vi "SVF System Simplified.vi"() -> ()   [LabVIEW 2012]
uses:
  <vilib>/addons/Control Design/_Model Construction/Data Typedefs.llb/CD Model Type.ctl
  <vilib>/addons/Control Design/_Model Construction/Model Typedefs.llb/CD Zero-Pole-Gain Model (MIMO).ctl
  <vilib>/addons/Control Design/_Model Construction/Model Typedefs.llb/CD General Elements.ctl
  <vilib>/addons/Control Design/_Model Construction/Model Typedefs.llb/CD Zero-Pole-Gain Model (SISO).ctl
  <vilib>/Simulation/Scripting/Companion Diagram/SimConfigNode/SimParams.ctl
  <vilib>/Simulation/Scripting/Companion Diagram/SimConfigNode/_simSolvers.ctl
  <vilib>/Simulation/Implementation/Shared/SIMSCR Execution Mode.ctl
  <vilib>/Platform/TimedLoop/XDataNode/timing_clust.ctl
  <vilib>/Platform/TimedLoop/XDataNode/nitl_modes.ctl
  <vilib>/Platform/TimedLoop/XDataNode/wakeup.ctl
  <vilib>/Simulation/Param Hierarchy/Typedefs/SIMPH Param Control Actions.ctl
  <vilib>/Simulation/Scripting/Editor Utilities/SIM subVI tag data.ctl
  <vilib>/Simulation/Scripting/Editor Utilities/SIM subVI execution type.ctl
  <vilib>/Simulation/Implementation/Shared/NILVSim_ParamChanged.vi
  <vilib>/Simulation/Implementation/Shared/NILVSim_FinishedLate.vi
  <vilib>/Simulation/ContinuousLinear/Implementation/NILVSim State Space.llb/SIM State Space Distributor (CD).vi
  <vilib>/Simulation/ContinuousLinear/Implementation/NILVSim Derivative.llb/SIM derivative (scalar).vi
  <vilib>/Simulation/ContinuousLinear/Implementation/NILVSim Transfer Function.llb/SIM Transfer Function Distributor (SISO).vi
  <vilib>/Simulation/ContinuousLinear/Implementation/NILVSim Transfer Function.llb/SIM Transfer Function Collector (SISO).vi
  <vilib>/Simulation/SignalDisplay/Implementation/NILVSim Time Waveform.llb/SIM Time Waveform (vector).vi
  <vilib>/Simulation/ContinuousLinear/Implementation/NILVSim State Space.llb/SIM State Space Collector (CD).vi
  <vilib>/Simulation/Implementation/Shared/SIM Fire Discrete SubVI.vi
  <vilib>/Simulation/Utility/Implementation/SIM Halt.vi
  <vilib>/Simulation/Implementation/Shared/NILVSim_Manager.vi
  <vilib>/Simulation/Implementation/Shared/NILVSim_FinalizeModel.vi
  <vilib>/Simulation/SignalArithmetic/Implementation/NILVSim Gain.llb/SIM Gain (scalar).vi
  <vilib>/Simulation/DiscreteLinear/Implementation/NILVSim Discrete State Space Buffered.llb/SIM Discrete State Space Distributor (CD).vi
  <vilib>/Simulation/SignalArithmetic/Implementation/NILVSim Gain.llb/SIM Gain (vector).vi
  <vilib>/Simulation/DiscreteLinear/Implementation/NILVSim Discrete State Space Buffered.llb/SIM Discrete State Space Collector (CD).vi
  <vilib>/Simulation/Implementation/Shared/SIM Fire Discrete SubVI (Core).vi
  <vilib>/addons/Control Design/_Dynamic Analysis/Dynamic Analysis.llb/Dynamic Analysis subVI/cd_Pole-Zero Map (State-Space).vi
  <vilib>/addons/Control Design/_Model Conversions/Model Type.llb/Model Conversion SubVI/cd_Convert State-Space to Zero-Pole-Gain Model.vi
  <vilib>/addons/Control Design/_Model Construction/Model Information.llb/Model Information SubVIs/cd_Verify If Discrete (State-Space).vi
  <vilib>/addons/Control Design/_Model Construction/Model Information.llb/Model Information SubVIs/cd_Check State Space Model.vi
  <vilib>/addons/Control Design/_Model Construction/Model Information.llb/Model Information SubVIs/cd_Verify Model Type (SS).vi
  <vilib>/addons/Control Design/_Dynamic Analysis/Dynamic Analysis.llb/Dynamic Analysis subVI/cd_Poles (State-Space).vi
  <vilib>/addons/Control Design/_Model Construction/Model Creation.llb/Model Creation SubVI/cd_Create State Space Model.vi
  <vilib>/addons/Control Design/_Model Conversions/Continuous and Discrete.llb/Continuous and Discrete SubVI/cd_Convert Continuous to Discrete (SS).vi
  <vilib>/Simulation/Implementation/Shared/SIM Unbundle Sim Info.vi
  <vilib>/Utility/error.llb/Clear Errors.vi
  <vilib>/Simulation/Implementation/Shared/NILVSim_GetModelError.vi
  <vilib>/Simulation/Implementation/Shared/SIM Bundle Sim Info.vi
  <vilib>/Simulation/Implementation/Shared/SIMSH Read Queue.vi
  <vilib>/Simulation/Implementation/Shared/NILVSim_Initialize.vi
  <vilib>/addons/Control Design/_Implementation/CD State Feedback Controller.vi
  <vilib>/addons/Control Design/_Implementation/CD State Feedback Controller (Single Output).vi
  <vilib>/Simulation/Utility/Implementation/NILVSim Get Time and IsAcceptedStep.vi
  Program Files/National Instruments/LabVIEW 2012/examples/Control and Simulation/Case Studies/Mechatronics/Inverted Pendulum/subVIs/Draw Linear Inverted Pendulum_sim.vi
  <vilib>/Simulation/Scripting/Companion Diagram/SimConfigNode/SimDog.xnode
  <vilib>/Platform/TimedLoop/XDataNode/XDataNode.xnode
  <vilib>/Simulation/Implementation/XNodeFramework/SimXNode/SimX.xnode
  <vilib>/addons/Control Design/_Implementation/NI_CD_Implementation.lvlib
  <vilib>/Simulation/ContinuousLinear/Implementation/NILVSim Transfer Function.llb/SIM Transfer Function (SISO).vi
  <vilib>/addons/Control Design/_Model Construction/NI_LinSys_Model Typedefs.lvlib
  <vilib>/addons/Control Design/_Model Construction/Model Typedefs.llb/CD State Space Model (MIMO).ctl
  <vilib>/Simulation/ContinuousLinear/Implementation/NILVSim State Space.llb/SIM State Space (CD).vi
  <vilib>/addons/Control Design/_State Feedback Control/NI_CD_State Feedback Control.lvlib
  <vilib>/addons/Control Design/_Model Construction/NI_LinSys_Model Creation.lvlib
  <vilib>/addons/Control Design/_Dynamic Analysis/NI_CD_Dynamic Analysis.lvlib
  <vilib>/addons/Control Design/_Model Conversions/NI_CD_Continuous and Discrete.lvlib
  <vilib>/addons/Control Design/_State-Space Analysis/NI_CD_State-Space Analysis.lvlib
  <vilib>/addons/Control Design/_Model Construction/NI_LinSys_Model Information.lvlib
  <vilib>/addons/Control Design/_Model Conversions/NI_CD_Model Type.lvlib
  <vilib>/Platform/TimedLoop/XDataNode/XDNodeRunTimeDep.lvlib
  <vilib>/Simulation/Implementation/Shared/NI_SIM_Implementation.lvlib
  <vilib>/Simulation/DiscreteLinear/Implementation/NILVSim Discrete State Space Buffered.llb/SIM Discrete State Space Buffered (CD).vi
  <vilib>/addons/Control Design/_Model Construction/NI_LinSys_Data Typedefs.lvlib
panel:
  in  "Input Signal (IMU)":dbl(slide) scale=0.0..10.0
  out "Controller Gain":dbl[](array[numeric])
  out "Waveform Plot":waveform(dbl)[](graph)
  in  "Inertia of pendulum (I)":dbl
  in  "Length to center of mass (l)":dbl
  in  "Kinetic friction of robot (b)":dbl
  in  "Mass of Rest (m)":dbl
  in  "Mass of Bottom Wheel (M)":dbl
  out "Pole-Zero Map":cluster{dbl[], dbl[]}[](graph)
  out "Zero-Pole-Gain Model":T1 {"zero-pole-gain(s)"."delay" format="%.4f"; "zero-pole-gain(s)"."Poles" format="%#.8g"; "zero-pole-gain(s)"."Zeros" format="%#.8g"; "zero-pole-gain(s)"."Gain" format="%#.8g"; "properties"."Sampling Time" format="%#.6p"; "properties"."Output Delays" format="%.4f"; "properties"."Input Delays" format="%.4f"}
  out "Static Gain Case?":bool
  out "Type of Model":T4 items=["Empty", "SISO", "SIMO", "MISO", "MIMO", "Undetermined"]
  out "Number of Outputs":i32
  out "Number of Inputs":i32
  out "Number of States":i32
  out "Sampling Time Required":dbl format="%.2f"
  out "Discrete?":bool
  out "Controllability Matrix":dbl[][](array[numeric])=[[1.0, 0.0, 6.0], [0.0, 1.0, -1.0], [0.0, 0.0, 0.0]] format="%.2f"
  out "Outputs":dbl[](array[numeric])
  out "Plot X and Theta":waveform(dbl)[](graph)=[{"t0"=timestamp(4.71 s since 1904-01-01), "dt"=1.0, "Y"=[-0.13996665083491025]}, {"t0"=timestamp(4.71 s since 1904-01-01), "dt"=1.0, "Y"=[-1.62298383744272e-05]}]
  in  "stop":bool
  in  "Tab Control":T5(tab)=enum."Controller"
  out "System Poles":cdb[](array[numeric])=[5.56510798020132+0.0i, -5.60409024766489+0.0i, -0.1428177325364319+0.0i, 0.0+0.0i] format="%#.2g"
  in  "Desired Poles":cdb[](array[numeric])=[-5.0+0.0i, -5.0+0.0i, -20.0+0.0i, -15.0+0.0i] format="%#.2g"
  out "Calculated Poles":cdb[](array[numeric])=[-19.999999999997662+0.0i, -15.000000000017264+0.0i, -4.999999999995586+4.2610378298679e-06i, -4.999999999995586-4.2610378298679e-06i] format="%#.2g"
  in  "Initial Conditions":T6
  in  "Set Point (m)":dbl(slide)=-0.14 scale=-0.2..0.2
  out "Feedback Gain (K)":dbl[](array[numeric])=[-168.36531967948676, -87.08873750117637, 222.70457028739702, 44.69540040141787]
  out "Boundary Reached":bool
  in  "Discrete Mode":bool=TRUE
  in  "A":dbl[][](array[numeric])=[[0.0, 1.0, 0.0, 0.0], [0.0, -0.1818, 2.6727, 0.0], [0.0, 0.0, 0.0, 1.0], [0.0, -0.4545, 31.1818, 0.0]] format="%#.2g"
  in  "B":dbl[][](array[numeric])=[[0.0], [1.8182], [0.0], [4.5455]] format="%#.2g"
  in  "C":dbl[][](array[numeric])=[[1.0, 0.0, 0.0, 0.0], [0.0, 0.0, 1.0, 0.0]] format="%#.2g"
  in  "D":dbl[][](array[numeric])=[[0.0], [0.0]] format="%#.2g"
  in  "Sampling Time (s)":dbl=0.1
  out "3D Picture Control":refnum<vi>(3d-picture)
  # "MODEL INFO"
  # "DISCRETE INFO"
  # "If you installed the LabVIEW Control Design Toolkit, you can design a controller by specifying the locations of the Desired Poles.\n\nOtherwise, click the Controller tab to specify the controller Feedback Gain."
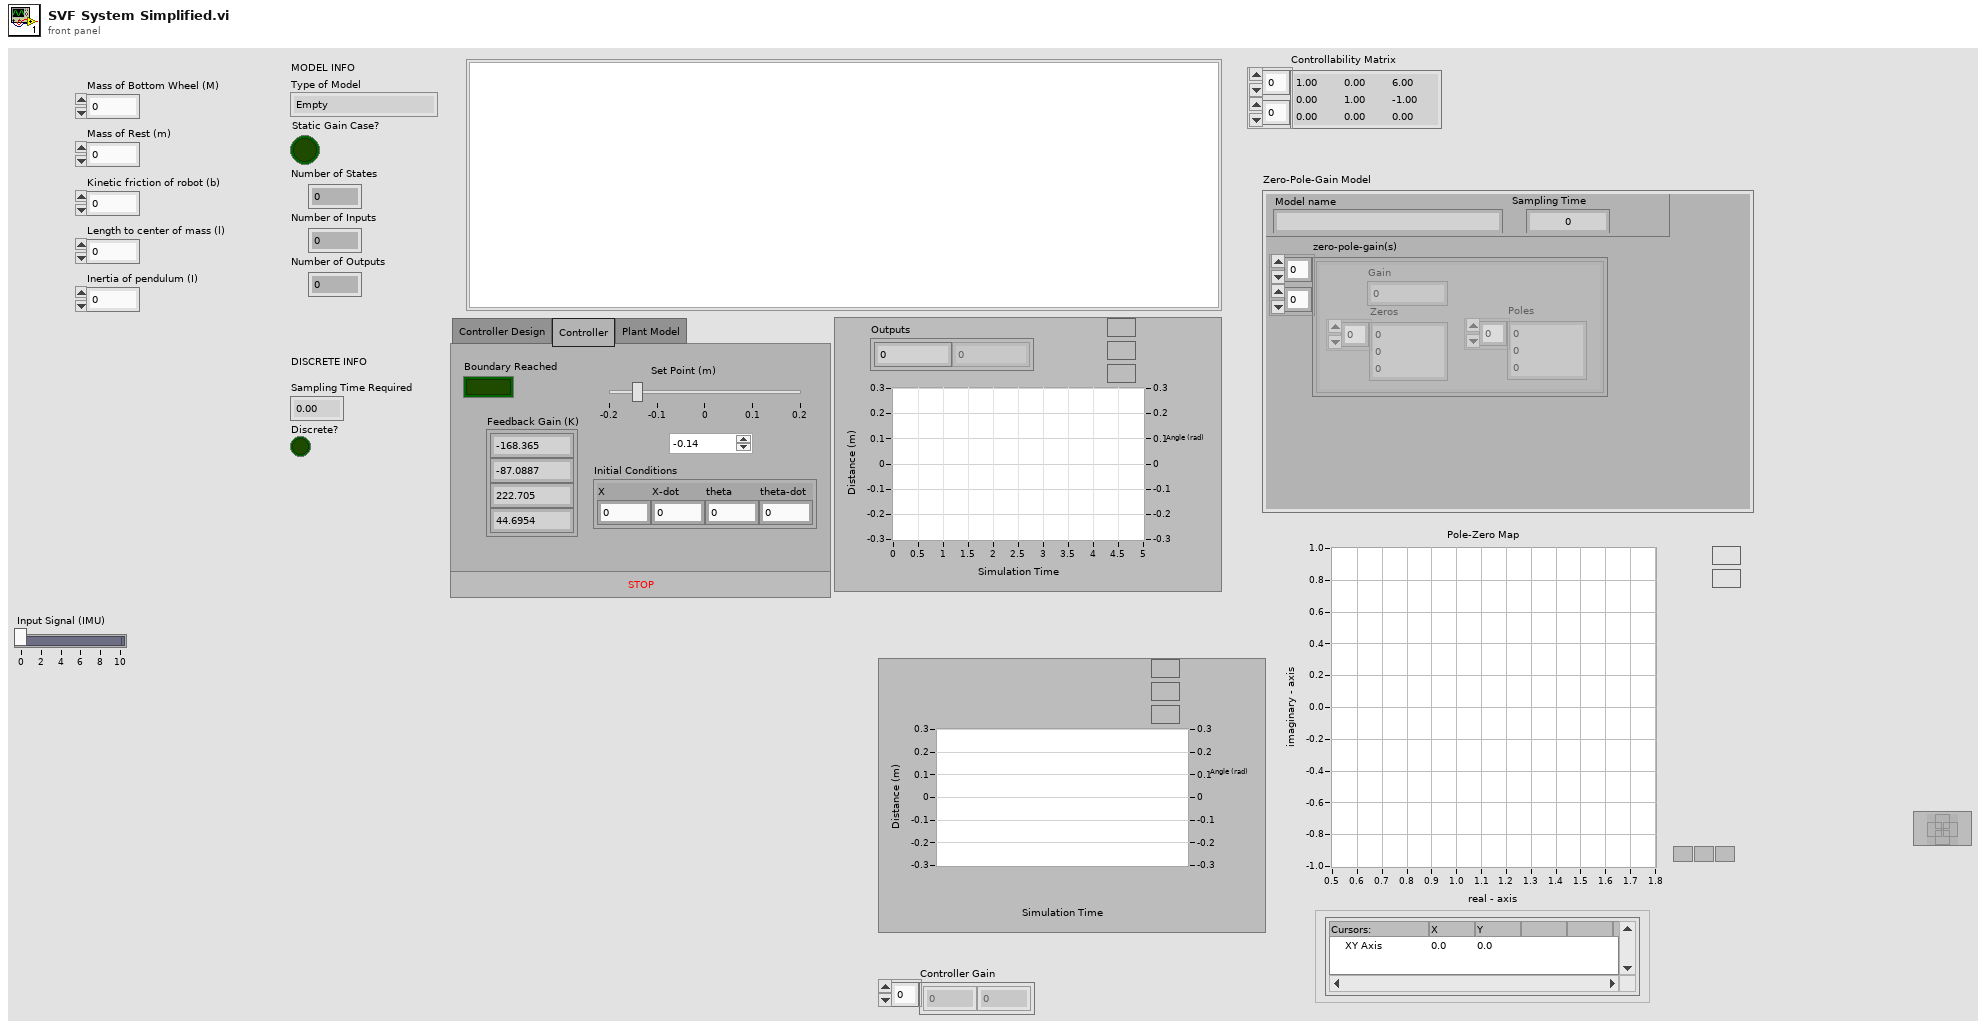
[diagram p1: front panel]
types:
  T1 = typedef "NI_LinSys_Model Typedefs.lvlib/CD Zero-Pole-Gain Model (MIMO).ctl" = cluster{"properties":T2, "zero-pole-gain(s)":T3[][]}
  T2 = typedef "NI_LinSys_Model Typedefs.lvlib/CD General Elements.ctl" = cluster{"Model name":string, "Input names":string[], "Output names":string[], "Input Delays":dbl[], "Output Delays":dbl[], "Sampling Time":dbl, "Notes":string}
  T3 = typedef "NI_LinSys_Model Typedefs.lvlib/CD Zero-Pole-Gain Model (SISO).ctl" = cluster{"Gain":dbl, "Zeros":cdb[], "Poles":cdb[], "delay":dbl}
  T4 = typedef "NI_LinSys_Data Typedefs.lvlib/CD Model Type.ctl" = u16
  T5 = enum32{"Controller Design", "Controller", "Plant Model"}
  T6 = cluster{"X":dbl, "X-dot":dbl, "theta":dbl, "theta-dot":dbl}
  T7 = typedef "NI_LinSys_Model Typedefs.lvlib/CD State Space Model (MIMO).ctl" = cluster{"properties":T2, "A":dbl[][], "B":dbl[][], "C":dbl[][], "D":dbl[][], "StateNames":string[], "Transport Delay":dbl[][]}
  T8 = typedef "SIMSCR Execution Mode.ctl" = enum16{"Simulate to Completion", "Single Time-Step Simulation (Fixed Step Only)"}
  T9 = typedef "XDNodeRunTimeDep.lvlib/timing_clust.ctl" = cluster{"Expected End [f-1]":u64, "Actual End [f-1]":u64, "Finished Late? [f-1]":bool, "Expected End [i-1]":u64, "Actual End [i-1]":u64, "Finished Late? [i-1]":bool, "Expected Start [i]":u64, "Actual Start [i]":u64, "Expected Start [f]":u64, "Actual Start [f]":u64, "Source Name":string, "Structure Name":string, "Period":i64, "Deadline":i64, "Offset":i64, "Start":i64, "Priority":i32, "Timeout":i32, "Mode":T10, "Wakeup Reason":T11, "Error":errorcluster, "Source Type":string, "Secondary Source Type":string, "Global End Time":u64, "Global Start Time":u64, "Frame Duration":u64, "Iteration Duration":u64, "Assigned CPU":i32, "I/O Scan Engine Mode":u32}
  T10 = typedef "XDNodeRunTimeDep.lvlib/nitl_modes.ctl" = enum32{"No Change", "Process missed periods, maintain original phase", "Discard missed periods, maintain original phase", "Process missed periods, ignore original phase", "Discard missed periods, ignore original phase"}
  T11 = typedef "XDNodeRunTimeDep.lvlib/wakeup.ctl" = enum32{"Normal", "Aborted", "Asynchronous wakeup", "Timing source error", "Timed loop error", "Timeout"}
  T12 = typedef "SIMPH Param Control Actions.ctl" = enum16{"get params", "set params"}
  T13 = typedef "SIM subVI tag data.ctl" = cluster{"period":dbl, "skew":dbl, "Simulation execution type":T14}
  T14 = typedef "SIM subVI execution type.ctl" = enum16{"Function call", "Discrete", "Continuous", "Initialization only", "Final step only"}
  T15 = typedef "SimParams.ctl" = cluster{"Initial Time (s)":dbl, "Final Time (s)":dbl, "Step Size (s)":dbl, "ODE Solver":T16, "Minimum Step Size (s)":dbl, "Maximum Step Size (s)":dbl, "Relative Tolerance":dbl, "Absolute Tolerance":dbl, "Software Timing":bool, "Initial Step Size (s)":dbl, "Automatic Fixed Step Size?":bool, "Automatic Discrete Step Size?":bool, "Discrete Step Size (s)":dbl, "Calculate using Time Step":bool, "Solver Wired?":bool, "Prev.Frm.Expected End":u64, "Prev.Frm.Actual End":u64, "Prev.Frm.Finished Late?":bool, "Prev.Iter.Expected End":u64, "Prev.Iter.Actual End":u64, "Prev.Iter.Finished Late?":bool, "Expected Iteration Start":u64, "Actual Iteration Start":u64, "Expected Frame Start":u64, "Actual Frame Start":u64, "Source Name":string, "Name":string, "Period":i64, "Deadline":i64, "Offset":i64, "Start":i64, "Priority":i32, "Timeout":i32, "Processor":i32, "Mode":enum32{"No Change", "Process missed periods, maintain original phase", "Discard missed periods, maintain original phase", "Process missed periods, ignore original phase", "Discard missed periods, ignore original phase"}, "Wakeup reason":enum32{"Normal", "Aborted", "Asynchronous wakeup", "Timing source error", "Timed loop error", "Timeout"}, "Error":errorcluster, "Source Type":string, "Secondary Source Type":string, "Global End Time":u64, "Global Start Time":u64, "Full Solver Reset":bool, "Execution Mode":T8, "Nan/Inf Check":bool, "Custom Solver Library":string, "Solver Is Variable":bool, "custom solver name":string, "Signal Collection Decimation":u32}
  T16 = typedef "_simSolvers.ctl" = enum16{"Runge-Kutta 1 (Euler)", "Runge-Kutta 2", "Runge-Kutta 3", "Runge-Kutta 4", "Runge-Kutta 23 (variable)", "Runge-Kutta 45 (variable)", "BDF (variable)", "Adams-Moulton (variable)", "Rosenbrock (variable)", "Discrete States Only", "SDIRK 4 (variable)", "Radau 5 (variable)", "Radau 9 (variable)", "Radau 13 (variable)", "Radau [Variable Order] (variable)", "Gear's Method (variable)", "Linearizer", "State Query", "Trim Eval", "Custom Solver"}
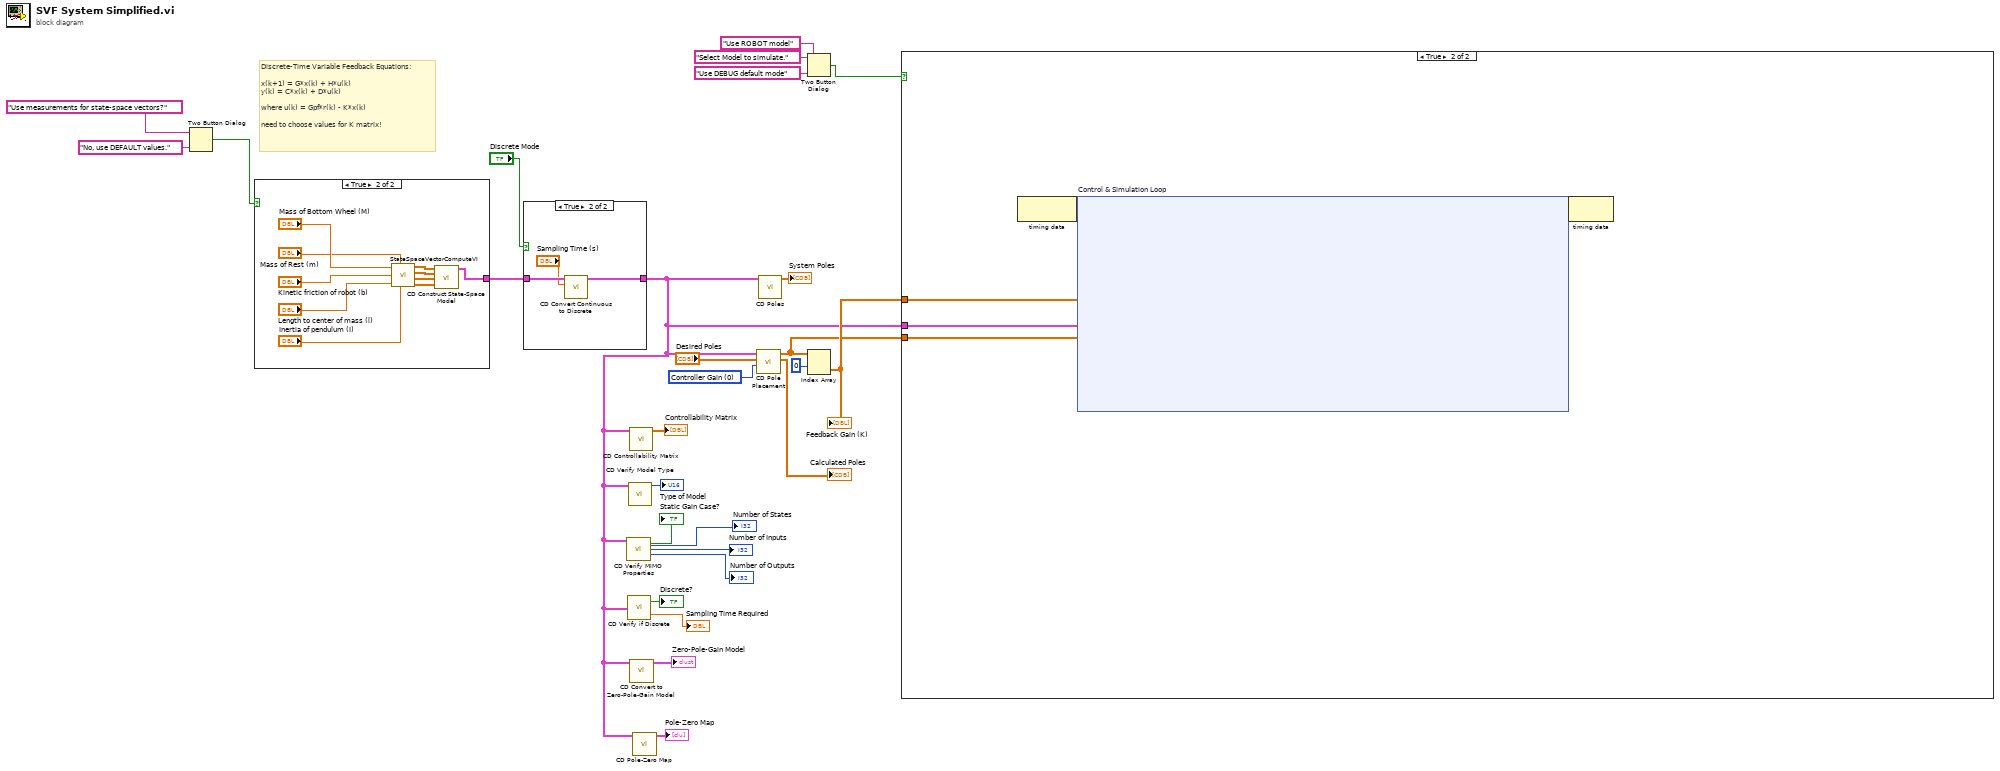
[diagram p0: block diagram]
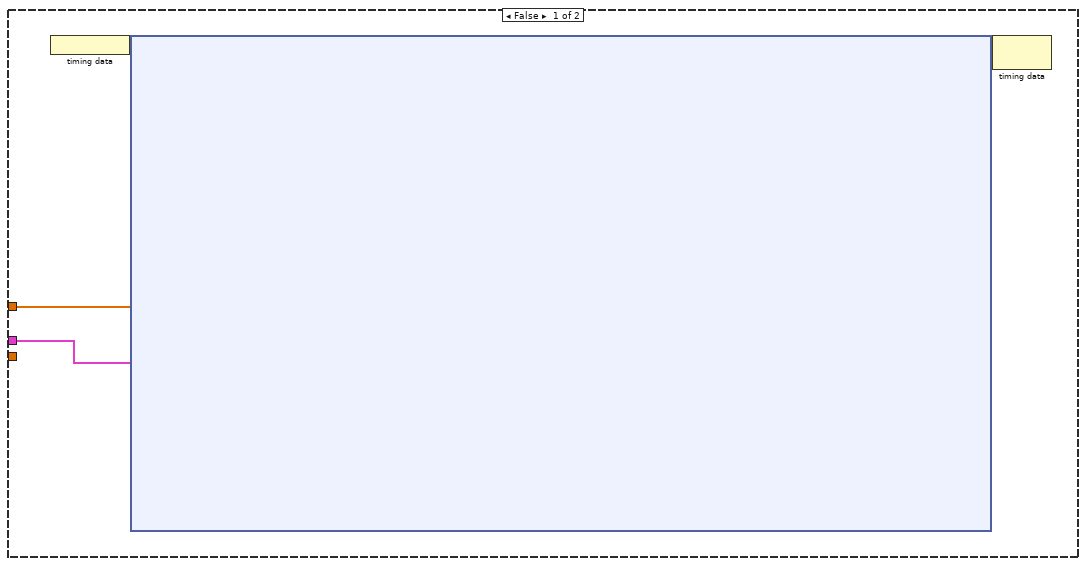
[diagram p2: hidden frame]
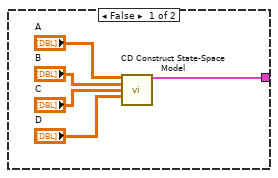
[diagram p3: hidden frame]
diagram:
  w27 = u16 0 items=["Controller Gain", "Observer Gain (Predictive)", "Observer Gain (Current)"] ("Gain Type")
  # "Discrete-Time Variable Feedback Equations:\n\nx(k+1) = G*x(k) + H*u(k)\ny(k) = C*x(k) + D*u(k)\n\nwhere u(k) = Gpf*r(k) - K*x(k)\n\nneed to choose values for K matrix!"
  n1 = Two Button Dialog(message="Use measurements for state-space vectors?", 1:"No, use DEFAULT values." ("F button name (\"Cancel\")")) -> (T button?=w9:bool)  [unwired: 1 in]
  n2 = case shown="True" w9 {
    tunnel: [w28 w33] -> w21
    frame False {
      n3 = call-poly <vilib>:"CD Construct State-Space Model.vi"("A"="A", "B"="B", "C"="C", "D"="D") -> ("State-Space Model"=w28:T7)  [unwired: 10 in, 1 out]
    }
    frame True {
      n4 = call "StateSpaceVectorComputeVI.vi"("Mass of Bottom Wheel (M)"="Mass of Bottom Wheel (M)", "Mass of Rest (m)"="Mass of Rest (m)", "Kinetic friction of robot (b)"="Kinetic friction of robot (b)", "Length to center of mass (l)"="Length to center of mass (l)", "Inertia of pendulum (I)"="Inertia of pendulum (I)") -> ("A"=w37:dbl[][], "B"=w36:dbl[][], "C"=w35:dbl[][], "D"=w34:dbl[][])
      n5 = call-poly <vilib>:"CD Construct State-Space Model.vi"("A"=w37, "B"=w36, "C"=w35, "D"=w34) -> ("State-Space Model"=w33:T7)  [unwired: 10 in, 1 out]
    }
  }
  n6 = case shown="True" "Discrete Mode" {
    tunnel: w21 -> [w43 w46]
    tunnel: [w43 w44] -> w2
    frame False {
    }
    frame True {
      n7 = call-poly <vilib>:"CD Convert Continuous to Discrete.vi"("Sampling Time (s)"="Sampling Time (s)", "Continuous State-Space Model"=w46) -> ("Discrete State-Space Model"=w44:T7)  [unwired: 7 in, 2 out]
    }
  }
  n8 = call-poly <vilib>:"CD Verify MIMO Properties.vi"("State-Space Model In"=w2) -> ("Static Gain Case?"=→"Static Gain Case?":bool, "Number of States"=→"Number of States":i32, "Number of Inputs"=→"Number of Inputs":i32, "Number of Outputs"=→"Number of Outputs":i32)  [unwired: 9 in, 2 out]
  n9 = call-poly <vilib>:"CD Verify if Discrete.vi"("State-Space Model"=w2) -> ("Discrete?"=→"Discrete?":bool, "Sampling Time"=→"Sampling Time Required":dbl)
  n10 = call-poly <vilib>:"CD Verify Model Type.vi"("State-Space Model"=w2) -> ("Type of Model"=→"Type of Model":T4)  [unwired: 9 in, 1 out]
  n11 = call <vilib>:"CD Controllability Matrix.vi"("State-Space Model"=w2) -> ("Controllability Matrix"=→"Controllability Matrix":dbl[][])  [unwired: 7 in, 3 out]
  n12 = call-poly <vilib>:"CD Convert to Zero-Pole-Gain Model.vi"("State-Space Model"=w2) -> ("Zero-Pole-Gain Model"=→"Zero-Pole-Gain Model":T1)  [unwired: 9 in, 1 out]
  n13 = call-poly <vilib>:"CD Pole-Zero Map.vi"("State-Space Model"=w2) -> ("Pole-Zero Map"=→"Pole-Zero Map":cluster{dbl[], dbl[]}[])  [unwired: 7 in, 3 out]
  n14 = call <vilib>:"CD Pole Placement.vi"("Gain Type"=w27, "Poles"="Desired Poles", "State-Space Model"=w2) -> ("Actual Poles"=→"Calculated Poles":cdb[], "Gain"=w1:dbl[][])  [unwired: 6 in, 1 out]
  n15 = call-poly <vilib>:"CD Poles.vi"("State-Space Model"=w2) -> ("Poles"=→"System Poles":cdb[])  [unwired: 9 in, 1 out]
  n16 = Two Button Dialog(message="Select Model to simulate.", 1:"Use DEBUG default mode" ("F button name (\"Cancel\")"), 2:"Use ROBOT model" ("T button name (\"OK\")")) -> (T button?=w6:bool)
  n17 = Index Array(array=w1, index (row)=0) -> (element=w22:dbl[])  [unwired: 1 in]
  "Feedback Gain (K)" <- w22
  n18 = case shown="True" w6 {
    tunnel: w22 -> [w48 w453]
    tunnel: w2 -> [w47 w452]
    tunnel: w1 -> [_ w451]
    frame False {
      n19 = node-c288() -> (w50:variant)
      n20 = node-c254 ("Simulation Loop")(w50, w47, w48) -> (w49:variant)
      n21 = node-c288(w49) -> ()  [unwired: 1 out]
    }
    frame True {
      n22 = node-c288() -> (w455:variant)  [unwired: 1 in]
      n23 = node-c254 "Control & Simulation Loop"(w455, w453, w452, w451) -> (w454:variant)
      n24 = node-c288(w454) -> ()  [unwired: 1 out]
    }
  }
